vi "load.vi"(8 "error in (no error)":errorcluster, 10 "functional":refnum<user-event>, 11 "interface in":refnum<class "interface.lvclass">=refnum) -> (0 "error out":errorcluster, 3 "interface out":refnum<class "interface.lvclass">)   [LabVIEW 2015, in "functional.lvlib" / "interface.lvclass"]
uses:
  interface.lvclass
  _controls/event_functional.ctl
  _controls/event_functional_command.ctl
  functional.lvlib
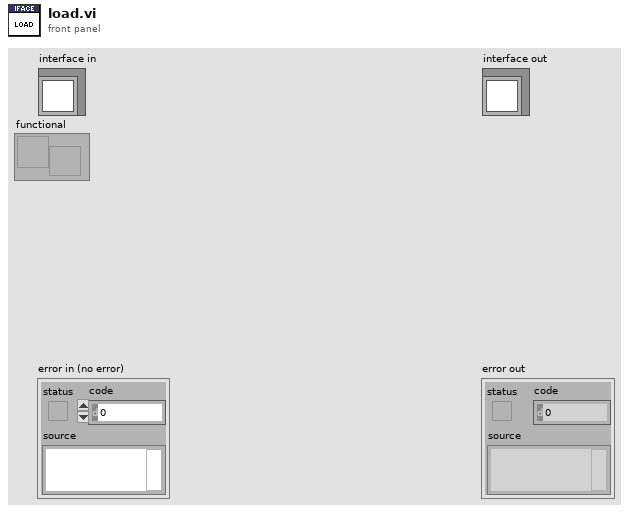
[diagram p1: front panel]
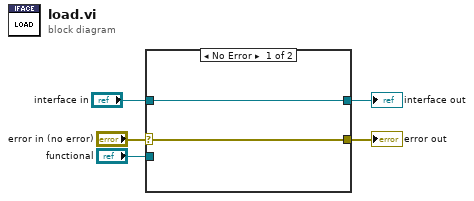
[diagram p0: block diagram]
diagram:
  n1 = case shown="No Error" "error in (no error)" {
    selector: "error in (no error)" -> [w6 w9]
    tunnel: [w6 w9] -> w4
    tunnel: [w7 w8] -> w2
    tunnel: "interface in" -> [w7 w8]
    tunnel: "functional" -> [_ _]
    frame No Error {
    }
    frame Error {
    }
  }
  "error out" <- w4
  "interface out" <- w2
